vi "ValveConrtoller.vi"(4 "INCOMMING SIGNAL":bool) -> (0 "OUTGOING SIGNAL":bool, 1 "CL":bool, 2 "OP":bool)   [LabVIEW 2010]
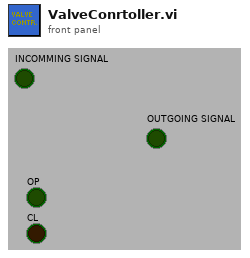
[diagram p1: front panel]
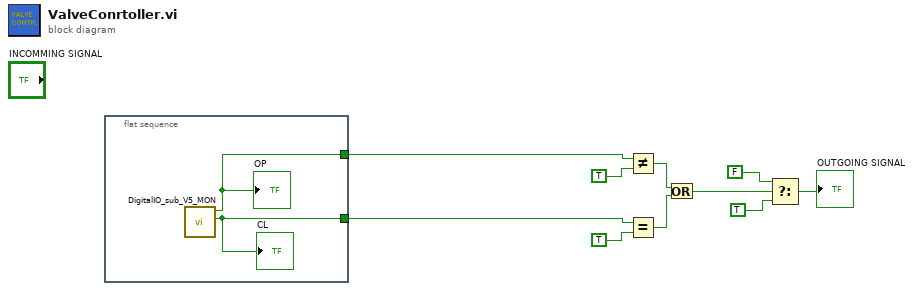
[diagram p0: block diagram]
diagram:
  n1 = flat-sequence {
    tunnel: [w12] -> w4
    tunnel: [w11] -> w10
    frame #0 {
      n2 = call "DigitalIO_sub_V5_MON.vi"() -> ("CL"=w11:bool, "OP"=w12:bool)  [unwired: 8 in]
      "CL" <- w11
      "OP" <- w12
    }
  }
  n3 = Not Equal?(x=w4, y=TRUE) -> (x != y?=w3:bool)
  n4 = Equal?(x=w10, y=TRUE) -> (x = y?=w2:bool)
  n5 = Or(x=w3, y=w2) -> (x .or. y?=w1:bool)
  n6 = Select(t=FALSE, s=w1, f=TRUE) -> (s? t:f=→"OUTGOING SIGNAL":bool)
